vi "ALTS-2015 LV2GBL Working Station Details.vi"(7 "Options":T1, 8 "error in":errorcluster) -> (0 "error out":errorcluster, 3 "Station  Enable Array":bool[](array[boolean]))   [LabVIEW 2013]
uses:
  Controls/ALTS-2015 LV2GBL Options.ctl
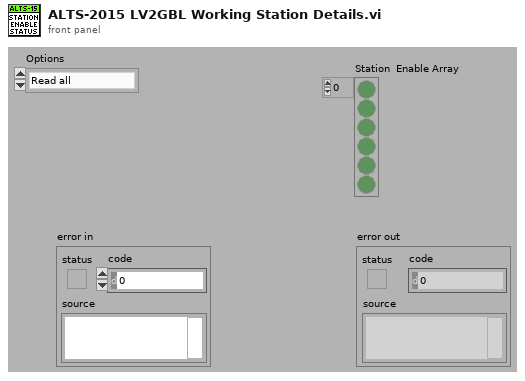
[diagram p1: front panel]
types:
  T1 = typedef "ALTS-2015 LV2GBL Options.ctl" = enum16{"Read all", "Write all"}
  T2 = typedef "ALTS-2015 INI Configuration Cluster.ctl" = cluster{"Application":cluster{"Rerun Count":i32, "Workorder No":string}, "Station Details":cluster{"Sensor Name 1":string, "Sensor Name 2":string, "Sensor Name 3":string, "Sensor Name 4":string, "Station1 Enable":bool, "Station2 Enable":bool, "Station3 Enable":bool, "Station4 Enable":bool}, "Database":cluster{"Database Connection Link":path, "Result Procedure":string, "User":string, "Password":string, "Prompt":bool, "Station 1 LT Result DB DSN Path":path, "Station 2 LT Result DB DSN Path":path, "Station 3 LT Result DB DSN Path":path, "Station 4 LT Result DB DSN Path":path, "AirLeakTestResult Procedure":string, "Serial Details Procedure":string}, "Simulation":cluster{"Simulate DAQ Hardware":bool, "Simulate Result DB Write":bool, "Simulate Scanner":bool, "Simulate OPC":bool, "Simulate Serial Details DB":bool, "Simulate Result DB":bool, "Simulate Scanner DB Path":path, "Simulate Serial Details DB Path":path, "Simulate Result DB Path":path}, "Barcode Scanner1":cluster{"Scanner IP":string, "Scanner Port":u16, "#Bytes to Read":i32}, "Barcode Scanner2":cluster{"Enabled?":bool, "Scanner IP":string, "Scanner Port":u16, "#Bytes to Read":i32}}
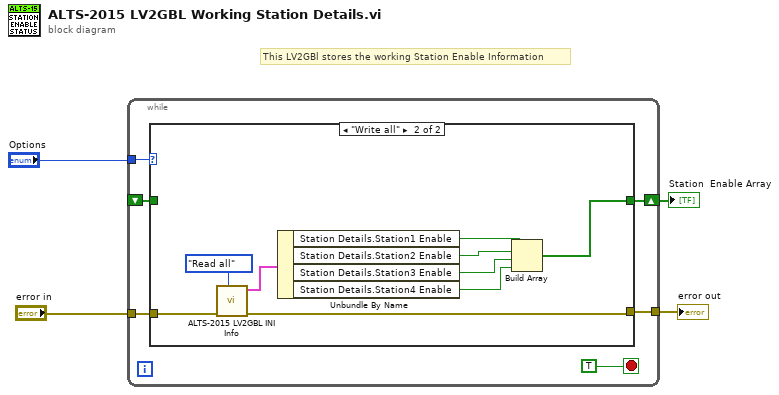
[diagram p0: block diagram]
diagram:
  # "This LV2GBl stores the working Station Enable Information"
  n1 = while {
    tunnel: "Options" -> [w9]
    tunnel: "error in" -> [w8]
    tunnel: [w7] -> w2
    shift-right: [w6] -> w1
    shift-left: _ -> [w5]
    stop <- TRUE stop-if-true
    n2 = case shown="\"Write all\"" w9 {
      tunnel: [w12 w20] -> w7
      tunnel: w8 -> [w12 w21]
      tunnel: [w11 w14] -> w6
      tunnel: w5 -> [w11 _]
      frame "Read all", Default {
      }
      frame "Write all" {
        n3 = call "ALTS-2015 LV2GBL INI Info.vi"("Options"=ALTS-2015_LV2GBL_Options."Read all", "error in"=w21) -> ("error out"=w20:errorcluster, "Configuration Cluster Out"=w19:T2)  [unwired: 8 in]
        n4 = Unbundle By Name(w19) -> ("Station Details.Station1 Enable"=w18:bool, "Station Details.Station2 Enable"=w17:bool, "Station Details.Station3 Enable"=w16:bool, "Station Details.Station4 Enable"=w15:bool)
        n5 = Build Array(w18, w17, w16, w15) -> (w14:bool[])
      }
    }
  }
  "error out" <- w2
  "Station  Enable Array" <- w1
